vi "Boolean Strings(lvlibp).vi"(8 "Enum":enum16{"List", "Add", "Remove"}(ring), 9 "Customer False Boolean Strings":string[](array[string]), 10 "Customer True Boolean Strings":string[](array[string])) -> (0 "Numeric":i32, 1 "False Boolean Strings":string[](array[string]), 2 "True Boolean Strings":string[](array[string]), 3 "Array":string[](array[string]))   [LabVIEW 2017, in "API String Arguments Support.lvlib"]
uses:
  API String Arguments Support.lvlib
  Boolean Strings.vi
  <userlib>/_NEVSTOP/Communicable State Machine(CSM)/Communicable State Machine.lvlib
  <userlib>/_NEVSTOP/Communicable State Machine(CSM)/_Shared/CSM Shared.lvlib
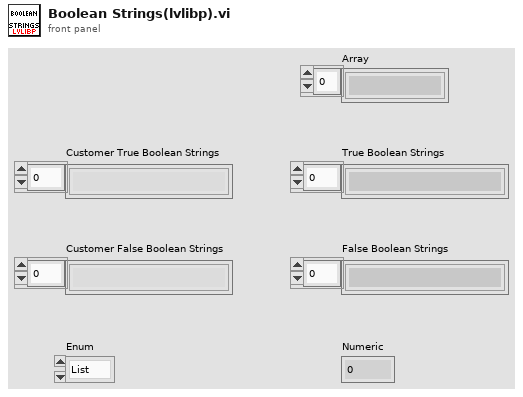
[diagram p1: front panel]
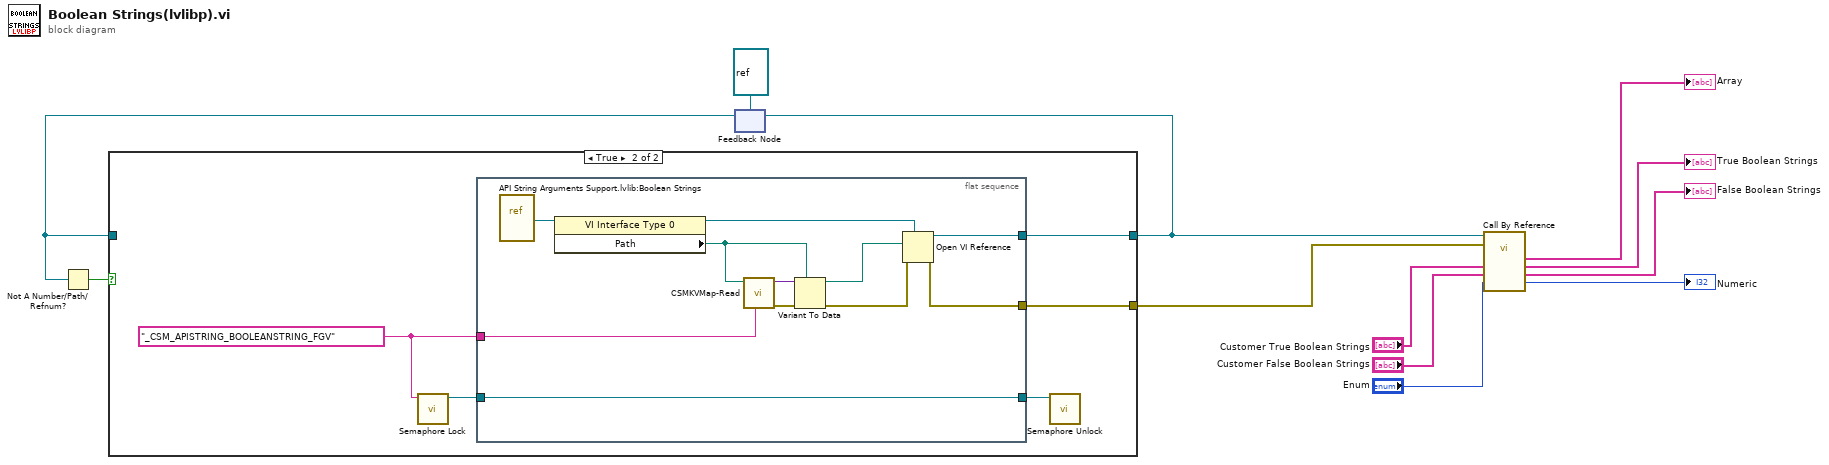
[diagram p0: block diagram]
diagram:
  n1 = feedback #1(refnum<vi> refnum) -> (w11:refnum<vi>)
  n2 = Not A Number/Path/Refnum?(number/path/refnum=w11) -> (NaN/Path/Refnum?=w12:bool)
  n3 = case shown="True" w12 {
    tunnel: [w13 w18] -> w9
    tunnel: w11 -> [w13 _]
    tunnel: [_ w17] -> w10
    frame False {
    }
    frame True {
      w14 = "_CSM_APISTRING_BOOLEANSTRING_FGV" ("name")
      n4 = call <userlib>:"Semaphore Lock.vi"("name"=w14) -> ("semaphore"=w15:refnum<queue>)  [unwired: 10 in]
      n5 = flat-sequence {
        tunnel: [w21] -> w18
        tunnel: [w24] -> w17
        tunnel: w14 -> [w20]
        tunnel: [w19] -> w16
        tunnel: w15 -> [w19]
        frame #0 {
          n6 = vi-ref "API String Arguments Support.lvlib:Boolean Strings.vi"() -> (w29:refnum<vi>)
          n7 = property class="VI Interface Type 0"(reference=w29) -> (reference out=w22:refnum<vi>, "Path"=w26:path)  [unwired: 1 in, 1 out]
          n8 = call <userlib>:"CSMKVMap-Read.vi"("name"=w20, "default value (empty variant)"=w26) -> ("Error out"=w28:errorcluster, "value"=w27:variant)  [unwired: 6 in]
          n9 = Variant To Data(error in=w28, type=w26, Variant=w27) -> (data=w25:path, error out=w23:errorcluster)
          n10 = Open VI Reference(type specifier VI Refnum (for type only)=w22, vi path=w25, error in (no error)=w23) -> (vi reference=w21:refnum<vi>, error out=w24:errorcluster)  [unwired: 3 in]
        }
      }
      n11 = call <userlib>:"Semaphore Unlock.vi"("semaphore"=w16) -> ()  [unwired: 11 in]
    }
  }
  n12 = feedback-in #1(w9) -> ()
  n13 = call-by-ref "?"(reference=w9, error in=w10, "Enum"="Enum", "Customer False Boolean Strings"="Customer False Boolean Strings", "Customer True Boolean Strings"="Customer True Boolean Strings") -> ("Numeric"=→"Numeric":i32, "False Boolean Strings"=→"False Boolean Strings":string[], "True Boolean Strings"=→"True Boolean Strings":string[], "Array"=→"Array":string[])  [unwired: 5 in, 2 out]
